vi "Read Discrete Inputs Response.vi"(8 "error in (no error)":errorcluster, 9 "Modbus Data Unit in":T1={"function"=1, "Data"=[]} {"function" items=["Read Discrete Inputs"=2, "Read Coils"=1, "Write Single Coil"=5, "Write Multiple Coils"=15, "Read Input Register"=4, "Read Holding Registers"=3, "Write Single Register"=6, "Write Multiple Registers"=16, "Read/Write Multiple Registers"=23, "Mask Write Register"=22, "Read FIFO Queue"=24, "Read File Record"=20, "Write File Record"=21, "Read Exception Status"=7, "Diagnostic"=8, "Get Com Event Counter"=11, "Get Com Event Log"=12, "Report Slave ID"=17, "Read Device Identification"=43]; "Data" format="%.0x"}) -> (0 "error out":errorcluster, 2 "data":bool[](array[boolean]))   [LabVIEW 2021, in "NI_modbus_upd.lvlib"]
doc: "Decodes the response for the read discrete inputs function."
uses:
  NI_modbus_upd.lvlib
  Ctl/MB Modbus Data Unit.ctl
  Modbus Data Unit (PDU)/Function.ctl
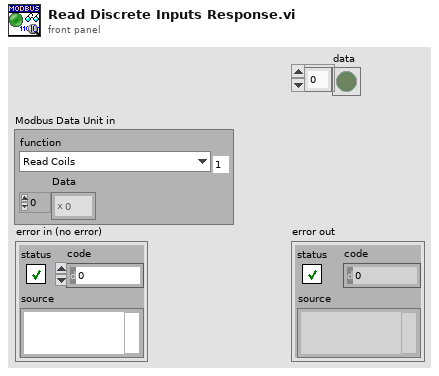
[diagram p1: front panel]
types:
  T1 = typedef "NI_modbus_upd.lvlib/MB Modbus Data Unit.ctl" = cluster{"function":T2, "Data":u8[]}
  T2 = typedef "NI_modbus_upd.lvlib/Function.ctl" = u8
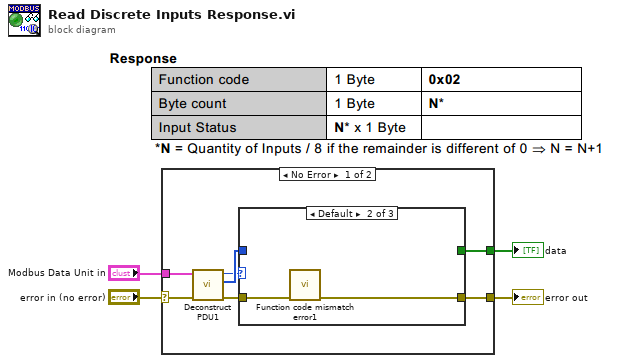
[diagram p0: block diagram]
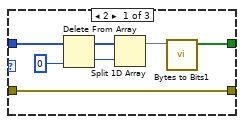
[diagram p2: hidden frame]
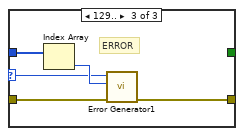
[diagram p3: hidden frame]
diagram:
  n1 = case shown="No Error" "error in (no error)" {
    selector: "error in (no error)" -> [w9 w26]
    tunnel: [w11 w26] -> w3
    tunnel: "Modbus Data Unit in" -> [w6 _]
    tunnel: [w10 _] -> w2
    frame No Error {
      n2 = call "Deconstruct PDU1.vi"("error in (no error)"=w9, "Modbus Data Unit in"=w6) -> ("error out"=w7:errorcluster, "data"=w8:u8[], "function"=w5:T2)  [unwired: 7 in]
      n3 = case shown="Default" w5 {
        selector: w5 -> [_ _ w21]
        tunnel: w7 -> [w16 w20 w22]
        tunnel: w8 -> [w18 _ w25]
        tunnel: [w16 w19 w24] -> w11
        tunnel: [w17 _ _] -> w10
        frame 2 {
          n4 = Delete From Array(array=w18, index=0) -> (deleted portion=w13:u8, array with subset deleted=w12:u8[])  [unwired: 1 in]
          n5 = Split 1D Array(array=w12, index=w13) -> (first subarray=w15:u8[])  [unwired: 1 out]
          n6 = call "Bytes to Bits1.vi"("bytes"=w15) -> ("bits"=w17:bool[])  [unwired: 10 in]
        }
        frame Default {
          n7 = call "Function code mismatch error1.vi"("error in (no error)"=w20) -> ("error out"=w19:errorcluster)  [unwired: 10 in]
        }
        frame 129.. {
          # "ERROR"
          n8 = Index Array(array=w25) -> (element=w23:u8)  [unwired: 1 in]
          n9 = call "Error Generator1.vi"("error in (no error)"=w22, "data return (error code)"=w23, "function return"=w21) -> ("error out"=w24:errorcluster)  [unwired: 8 in]
        }
      }
    }
    frame Error {
    }
  }
  "error out" <- w3
  "data" <- w2
